vi "VariantToLithoData.vi"(11 "Lithography Data In":T2(array[cluster])) -> (3 "Lithography Data Out":T3(array[cluster]))   [LabVIEW 2020]
uses:
  <userlib>/LevyLab/Relay Box/Type_defs/Resistor--enum.ctl
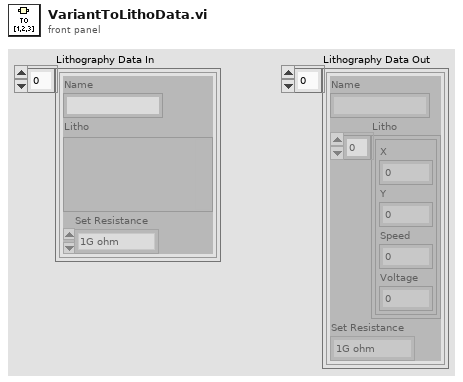
[diagram p1: front panel]
types:
  T1 = typedef "Resistor--enum.ctl" = enum16{"open", "discharge tip", "0 ohms", "100k ohm", "10M ohm", "1G ohm"}
  T2 = cluster{"Name":string, "Litho":variant, "Set Resistance":T1}[]
  T3 = cluster{"Name":string, "Litho":cluster{"X":dbl, "Y":dbl, "Speed":dbl, "Voltage":dbl}[], "Set Resistance":T1}[]
  T4 = cluster{"Name":string, "Litho":cluster{"X":dbl, "Y":dbl, "Speed":dbl, "Voltage":dbl}[], "Set Resistance":T1}
  T5 = cluster{"X":dbl, "Y":dbl, "Speed":dbl, "Voltage":dbl}[]
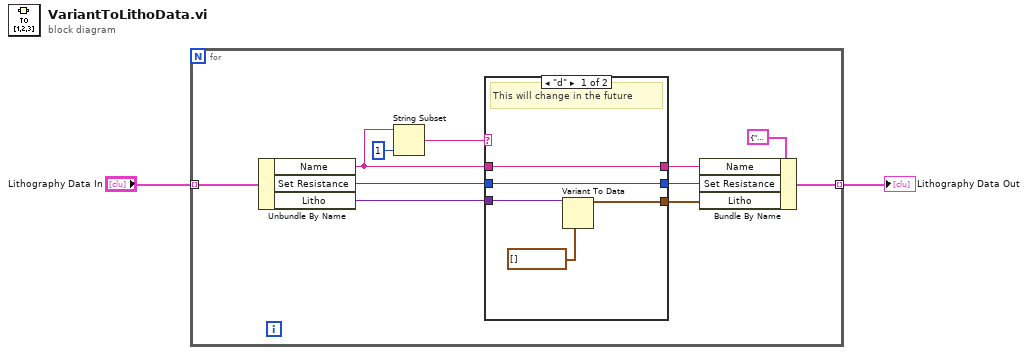
[diagram p0: block diagram]
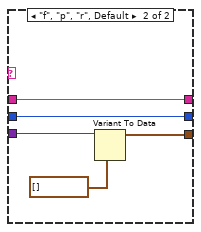
[diagram p2: hidden frame]
diagram:
  n1 = for {
    tunnel: [w6] -> w2 mode=indexing
    tunnel: "Lithography Data In" -> [w13] mode=indexing
    n2 = Unbundle By Name(w13) -> ("Name"=w8:string, "Set Resistance"=w9:T1, "Litho"=w10:variant)
    n3 = String Subset(string=w8, length (rest)=1 ("length (rest)")) -> (substring=w11:string)  [unwired: 1 in]
    n4 = case shown="\"d\"" w11 {
      tunnel: w10 -> [w18 w23]
      tunnel: w9 -> [w16 w21]
      tunnel: [w16 w21] -> w4
      tunnel: w8 -> [w15 w20]
      tunnel: [w15 w20] -> w5
      tunnel: [w14 w19] -> w3
      frame "d" {
        # "This will change in the future"
        n5 = Variant To Data(type=T5 [] ("Litho"), Variant=w18) -> (data=w14:T5)  [unwired: 1 in, 1 out]
      }
      frame "f", "p", "r", Default {
        n6 = Variant To Data(type=T5 [] ("Litho"), Variant=w23) -> (data=w19:T5)  [unwired: 1 in, 1 out]
      }
    }
    n7 = Bundle By Name(cluster=T4 {"Name"="", "Litho"=[], "Set Resistance"=enum."1G ohm"} ("Pattern Data"), "Name"=w5, "Set Resistance"=w4, "Litho"=w3) -> (w6:T4)
  }
  "Lithography Data Out" <- w2
